vi "loops_local_var.vi"() -> ()   [LabVIEW 2022 SP3]
panel:
  out "millisecond timer value 2":u32
  out "millisecond timer value":u32
  in  "stop":bool
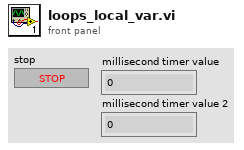
[diagram p1: front panel]
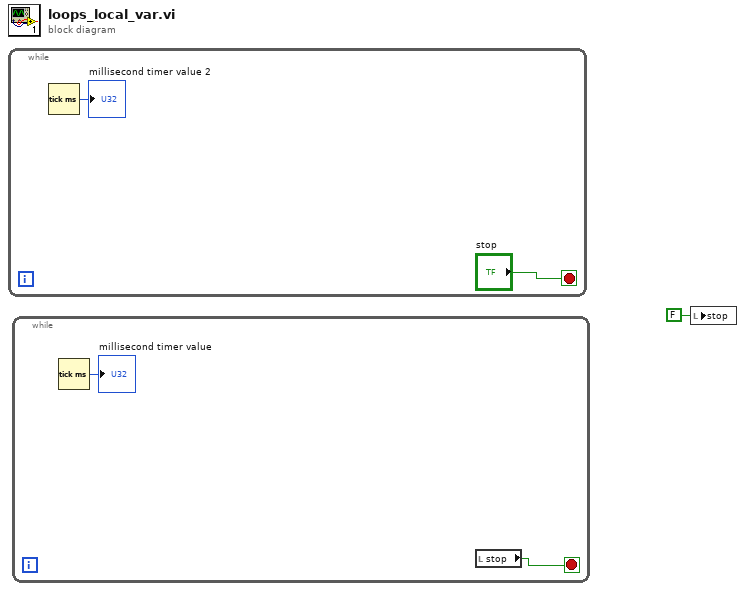
[diagram p0: block diagram]
diagram:
  n1 = while {
    stop <- "stop" stop-if-true
    n2 = Tick Count (ms)() -> (millisecond timer value=→"millisecond timer value 2":u32)
  }
  n3 = while {
    stop <- w5 stop-if-true
    n4 = Tick Count (ms)() -> (millisecond timer value=→"millisecond timer value":u32)
    n5 = local read "stop"() -> (w5:bool)
  }
  n6 = local write "stop"(FALSE ("stop")) -> ()
